vi "Practica10_Dobleservo.vi"() -> ()   [LabVIEW 2015]
uses:
  <vilib>/LabVIEW Interface for Arduino/LabVIEW Interface for Arduino.lvlib
panel:
  in  "Numebro de servo":u8=1
  in  "stop":bool
  out "Control 2":dbl(knob) scale=0.0..10.0
  in  "Angulo":dbl(knob) scale=0.0..180.0
  in  "Barrido":u8(knob) scale=0.0..180.0
  in  "Velocidad":u8(knob) scale=0.0..10.0
  out "Control 1":dbl(knob) scale=0.0..10.0
  # "Control de Servos"
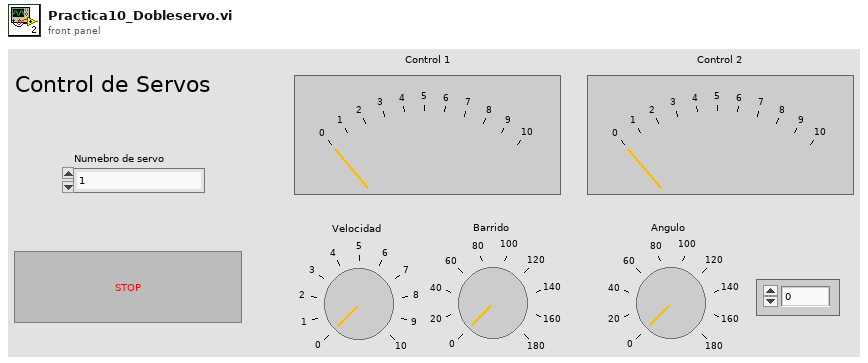
[diagram p1: front panel]
types:
  T1 = typedef "LabVIEW Interface for Arduino.lvlib/Arduino Resource.ctl" = cluster{"VISA resource":refnum<visa-resource-name>, "Board Type":T2, "Connection Type":enum8{"USB / Serial"}, "Bytes Per Packet (15)":u8}
  T2 = typedef "LabVIEW Interface for Arduino.lvlib/Board Type.ctl" = enum16{"Uno", "Dimuelanove w/Atmega 328", "Mega 2560"}
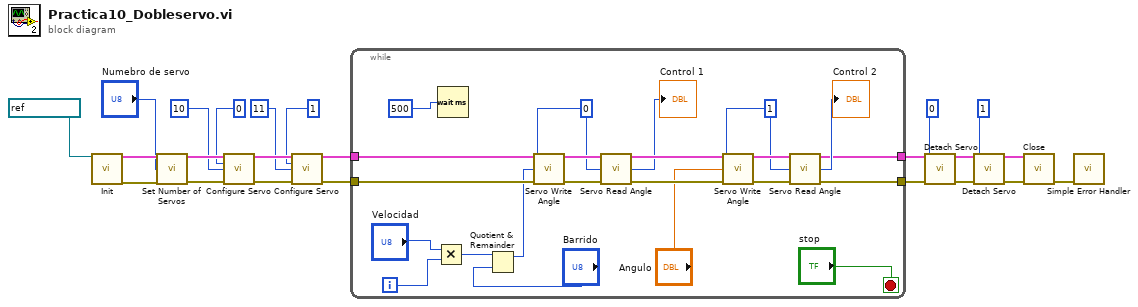
[diagram p0: block diagram]
diagram:
  n1 = call <vilib>:"Init.vi"("VISA resource"=refnum<visa-resource-name> "COM7") -> ("Arduino Resource"=w22:T1, "error out"=w23:errorcluster)  [unwired: 17 in]
  n2 = call <vilib>:"Set Number of Servos.vi"("Arduino Resource"=w22, "Number Of Servos (1)"="Numebro de servo", "error in"=w23) -> ("Arduino Resource"=w21:T1, "error out"=w18:errorcluster)  [unwired: 11 in]
  n3 = call <vilib>:"Configure Servo.vi"("Arduino Resource"=w21, "Servo Number (0)"=u8 0, "DIO Pin (2)"=u8 10, "error in"=w18) -> ("Arduino Resource"=w20:T1, "error out"=w17:errorcluster)  [unwired: 10 in]
  n4 = call <vilib>:"Configure Servo.vi"("Arduino Resource"=w20, "Servo Number (0)"=u8 1, "DIO Pin (2)"=u8 11, "error in"=w17) -> ("Arduino Resource"=w19:T1, "error out"=w16:errorcluster)  [unwired: 10 in]
  n5 = while {
    tunnel: w19 -> [w45]
    tunnel: w16 -> [w41]
    tunnel: [w27] -> w8
    tunnel: [w26] -> w5
    i -> [w36]
    stop <- "stop" stop-if-true
    w29 = u8 1 ("Servo Number")
    w30 = u8 0 ("Servo Number")
    n6 = Multiply(x="Velocidad", y=w36) -> (x*y=w35:i32)
    n7 = Wait (ms)(milliseconds to wait=u32 500) -> ()  [unwired: 1 out]
    n8 = Quotient & Remainder(x=w35, y="Barrido") -> (x-y*floor(x/y)=w33:i32)  [unwired: 1 out]
    n9 = call <vilib>:"Servo Write Angle.vi"("Arduino Resource"=w45, "Servo Number"=w30, "Angle (Degrees)"=w33, "error in"=w41) -> ("Arduino Resource"=w44:T1, "error out"=w40:errorcluster)  [unwired: 10 in]
    n10 = call <vilib>:"Servo Read Angle.vi"("Arduino Resource"=w44, "Servo Number"=w30, "error in"=w40) -> ("Arduino Resource"=w43:T1, "Angle (Degrees)"=→"Control 1":u8, "error out"=w39:errorcluster)  [unwired: 10 in]
    n11 = call <vilib>:"Servo Write Angle.vi"("Arduino Resource"=w43, "Servo Number"=w29, "Angle (Degrees)"="Angulo", "error in"=w39) -> ("Arduino Resource"=w42:T1, "error out"=w38:errorcluster)  [unwired: 10 in]
    n12 = call <vilib>:"Servo Read Angle.vi"("Arduino Resource"=w42, "Servo Number"=w29, "error in"=w38) -> ("Arduino Resource"=w27:T1, "Angle (Degrees)"=→"Control 2":u8, "error out"=w26:errorcluster)  [unwired: 10 in]
  }
  n13 = call <vilib>:"Detach Servo.vi"("Arduino Resource"=w8, "Servo Number"=u8 0, "error in"=w5) -> ("Arduino Resource"=w7:T1, "error out"=w4:errorcluster)  [unwired: 11 in]
  n14 = call <vilib>:"Detach Servo.vi"("Arduino Resource"=w7, "Servo Number"=u8 1, "error in"=w4) -> ("Arduino Resource"=w6:T1, "error out"=w3:errorcluster)  [unwired: 11 in]
  n15 = call <vilib>:"Close.vi"("Arduino Resource"=w6, "error in"=w3) -> ("error out"=w9:errorcluster)  [unwired: 13 in]
  n16 = call <vilib>:"Simple Error Handler.vi"("error in (no error)"=w9) -> ()  [unwired: 4 in, 5 out]
